vi "Get Width.vi"(8 "error in":errorcluster, 11 "Generic Image in":refnum<class "Generic Image.lvclass">) -> (0 "error out":errorcluster, 2 "Width":i32, 3 "Generic Image out":refnum<class "Generic Image.lvclass">)   [LabVIEW 2025, in "Generic Image.lvclass"]
uses:
  Generic Image.lvclass
  Generic Image.lvclass/Generic Image.ctl
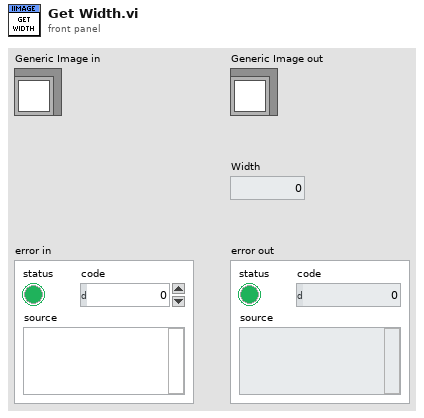
[diagram p1: front panel]
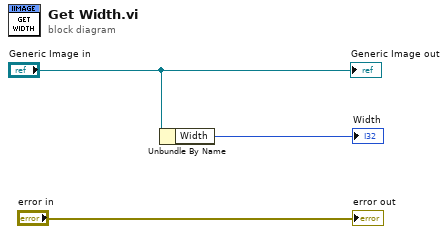
[diagram p0: block diagram]
diagram:
  n1 = Unbundle By Name("Generic Image in") -> ("Width"=→"Width":i32)
  "Generic Image out" <- "Generic Image in"
  "error out" <- "error in"
